vi "VD-test.vi"() -> ()   [LabVIEW 2020, in "VD-LV-LiteVNA.lvclass"]
uses:
  VD-LV-LiteVNA.lvclass
  VD-settings.ctl
  VD-data_req.ctl
  hardware-protocol/serial/HP-S-data.ctl
  VD-device_info.ctl
  VD-connection_settings.ctl
  hardware-protocol/serial/HP-S-baudrate.ctl
  VD-session_info.ctl
  VD-data_read_status.ctl
  VD-settings_status.ctl
  VD-settingsEasy.ctl
  VD-sampleSize.ctl
  VD-LV-LiteVNA.lvclass/VD-LV-LiteVNA.ctl
  hardware-protocol/serial/HP-S-Serial.lvclass
panel:
  out "current time":timestamp
  in  "Tab Control":enum32{"Main", "Bonus"}(tab)
  in  "Set Settings":bool
  in  "Settings":T1
  out "Settings status":T2
  in  "Set Settings easy":bool
  in  "settings":T3={"Start [hz]"=1000000, "Stop [hz]"=5000000, "sampleSize"=101} {"sampleSize" items=["101"=101, "201"=201, "401"=401, "601"=601, "801"=801, "1001"=1001]; "Stop [hz]" format="%.0p"; "Start [hz]" format="%.0p"}
  in  "Get Settings":bool
  in  "Get Data":bool
  in  "data req":T5
  out "read buffer":T6 format="%x"
  out "size(s)":i32
  in  "get device settings":bool
  out "device info":T7
  in  "raw request":bool
  in  "raw write buffer":T6 format="%x"
  out "read bufferraw":T6 format="%x"
  out "size(s) raw":i32
  in  "read back?":bool
  out "Get Settings status":T2
  out "data status":T8
  out "Valid Data?":bool
  out "size":i32
  out "XY Graph":cluster{u64[], dbl[]}[](graph)
  in  "get set":bool
  out "session info":T9 {"last get" format="%x"; "last set" format="%x"}
  out "Remaining Bytes":u32
  out "Emtpied size(s)":i32
  out "Emtpied buffer":T6 format="%x"
  in  "Empty Buffer":bool
  out "error IO":errorcluster
  in  "connection settings":T10={"Com"="", "baud rate (9600)"=38400} {"baud rate (9600)" items=["75"=75, "110"=110, "134"=134, "150"=150, "300"=300, "600"=600, "1200"=1200, "1800"=1800, "2400"=2400, "4800"=4800, "7200"=7200, "9600"=9600, "14400"=14400, "19200"=19200, "28800"=28800, "38400"=38400, "56000"=56000, "57600"=57600, "115200"=115200, "128000"=128000, "230400"=230400]}
  out "error out":errorcluster
  in  "Free Run":bool
  in  "Disconnect":bool
  in  "Stop":bool
  in  "Connect":bool
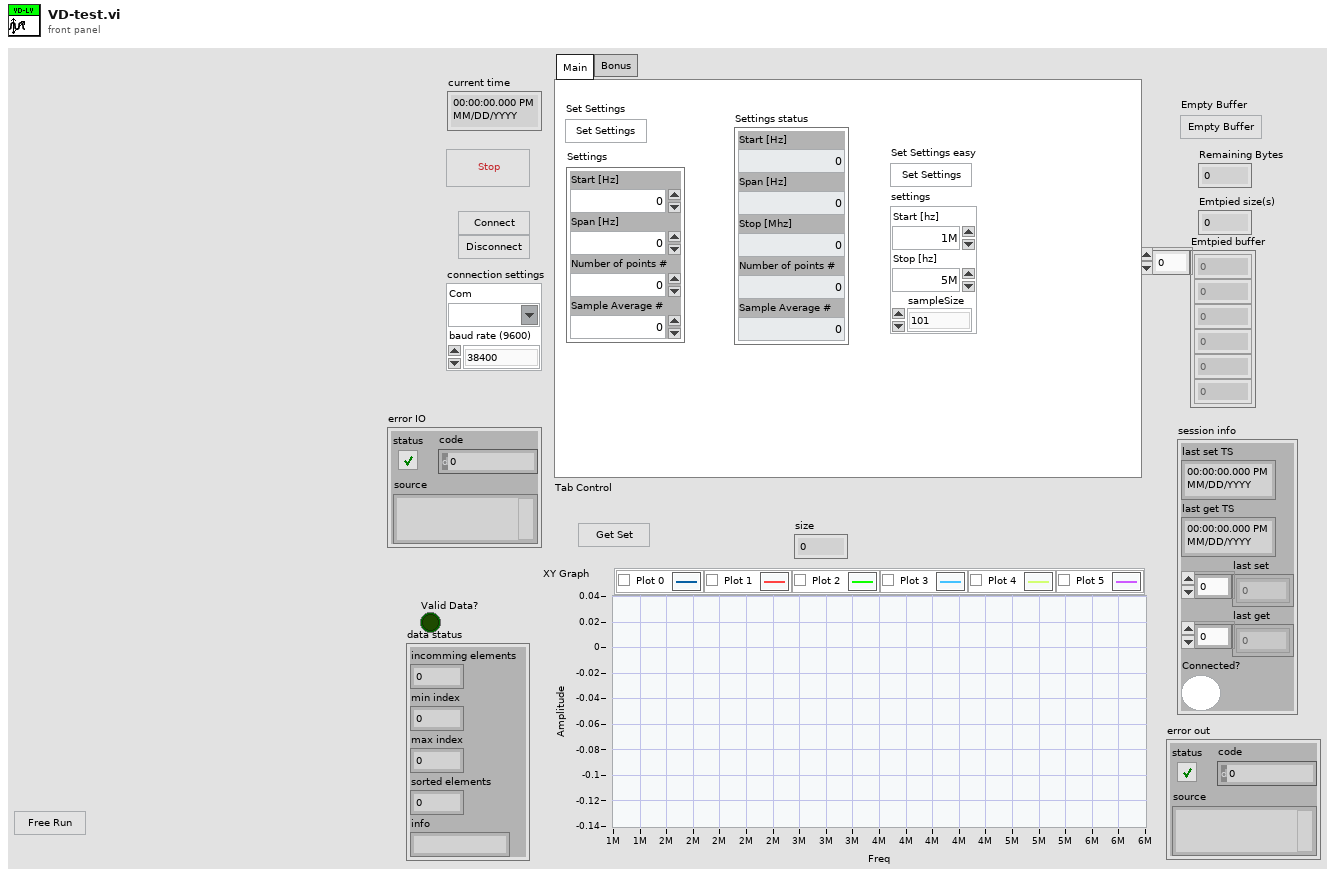
[diagram p1: front panel]
types:
  T1 = typedef "VD-LV-LiteVNA.lvclass/VD-settings.ctl" = cluster{"Start [Hz]":u64, "Span [Hz]":u64, "Number of points #":u16, "Sample Average #":u16}
  T2 = typedef "VD-LV-LiteVNA.lvclass/VD-settings_status.ctl" = cluster{"Start [Hz]":u64, "Span [Hz]":u64, "Stop [Mhz]":u64, "Number of points #":u16, "Sample Average #":u16}
  T3 = typedef "VD-LV-LiteVNA.lvclass/VD-settingsEasy.ctl" = cluster{"Start [hz]":u64, "Stop [hz]":u64, "sampleSize":T4}
  T4 = typedef "VD-LV-LiteVNA.lvclass/VD-sampleSize.ctl" = u16
  T5 = typedef "VD-LV-LiteVNA.lvclass/VD-data_req.ctl" = cluster{"datasize":u8}
  T6 = typedef "HP-S-Serial.lvclass/HP-S-data.ctl" = u8[]
  T7 = typedef "VD-LV-LiteVNA.lvclass/VD-device_info.ctl" = cluster{"ID":u8}
  T8 = typedef "VD-LV-LiteVNA.lvclass/VD-data_read_status.ctl" = cluster{"incomming elements":i32, "min index":u16, "max index":u16, "sorted elements":i32, "info":string}
  T9 = typedef "VD-LV-LiteVNA.lvclass/VD-session_info.ctl" = cluster{"last set TS":timestamp, "last get TS":timestamp, "last set":T6, "last get":T6, "Connected?":bool}
  T10 = typedef "VD-LV-LiteVNA.lvclass/VD-connection_settings.ctl" = cluster{"Com":refnum<visa-resource-name>, "baud rate (9600)":T11}
  T11 = typedef "HP-S-Serial.lvclass/HP-S-baudrate.ctl" = u32
  T12 = typedef "VD-LV-LiteVNA.lvclass/VD-VNA_data.ctl" = cluster{"S1":cdb[], "S11":cdb[], "S21":cdb[], "Frequency":u64[]}
  T13 = typedef "VD-LV-LiteVNA.lvclass/VD-graph_data.ctl" = cluster{u64[], dbl[]}[]
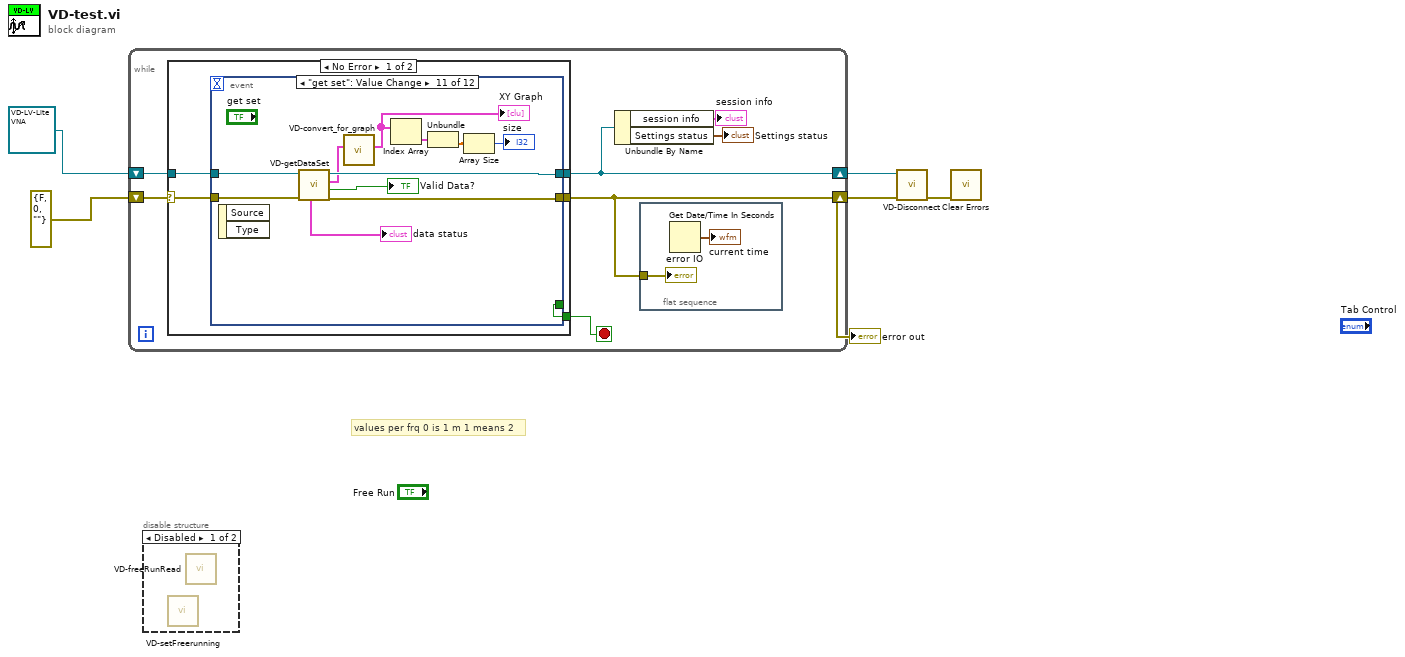
[diagram p0: block diagram]
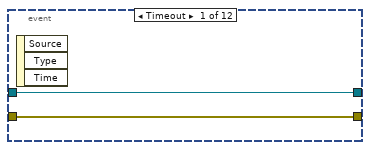
[diagram p2: hidden frame]
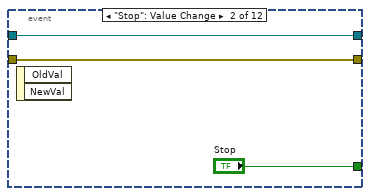
[diagram p3: hidden frame]
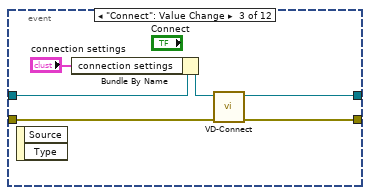
[diagram p4: hidden frame]
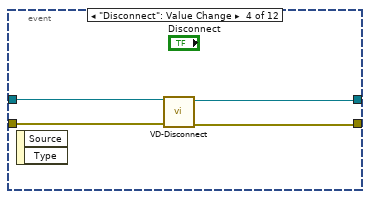
[diagram p5: hidden frame]
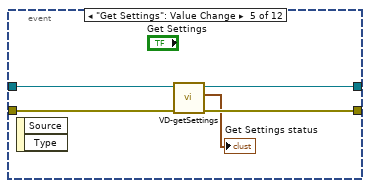
[diagram p6: hidden frame]
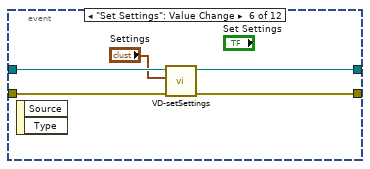
[diagram p7: hidden frame]
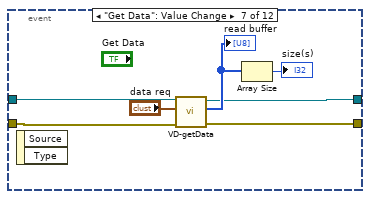
[diagram p8: hidden frame]
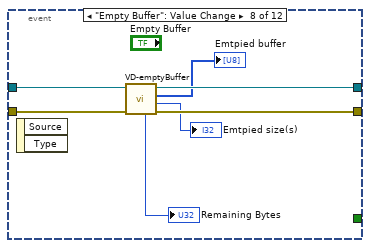
[diagram p9: hidden frame]
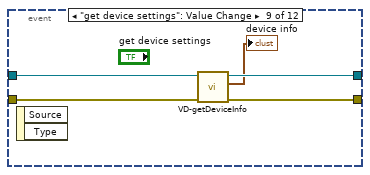
[diagram p10: hidden frame]
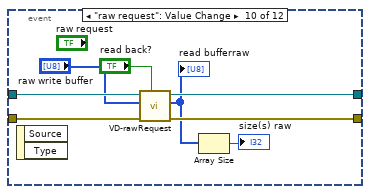
[diagram p11: hidden frame]
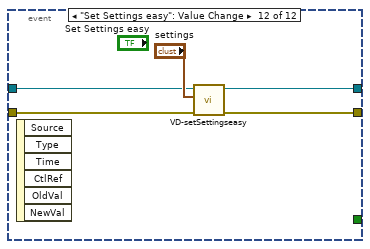
[diagram p12: hidden frame]
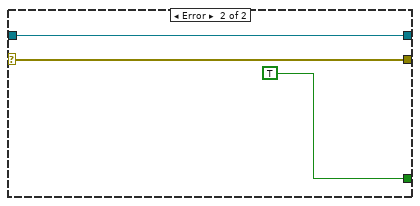
[diagram p13: hidden frame]
diagram:
  # "values per frq 0 is 1 m 1 means 2"
  n1 = while {
    shift-right: [w10] -> w3
    shift-left: errorcluster {"status"=FALSE, "code"=0, "source"=""} ("error IO") -> [w11]
    shift-right: [w8] -> w2
    shift-left: refnum<class "VD-LV-LiteVNA.lvclass"> refnum ("VD-LV-LiteVNA out") -> [w9]
    stop <- w12 stop-if-true
    n2 = case shown="No Error" w11 {
      selector: w11 -> [w19 w88]
      tunnel: [w17 TRUE] -> w12
      tunnel: [w18 w88] -> w10
      tunnel: w9 -> [w16 w89]
      tunnel: [w15 w89] -> w8
      frame No Error {
        n3 = event shown="[10] \"get set\": Value Change" {
          selector: _ -> [_ _ _ _ _ _ _ _ _ _ _ _]
          dyn-events: _ -> [_ _ _ _ _ _ _ _ _ _ _ _]
          timeout: _ -> [_ _ _ _ _ _ _ _ _ _ _ _]
          tunnel: w19 -> [w21 w23 w30 w33 w39 w43 w50 w57 w62 w70 w81 w85]
          tunnel: [w21 w23 w27 w32 w36 w41 w45 w56 w61 w67 w80 w83] -> w18
          tunnel: [_ "Stop" _ _ _ _ _ _ _ _ _ _] -> w17
          tunnel: w16 -> [w20 w22 w29 w34 w38 w44 w51 w58 w63 w71 w82 w86]
          tunnel: [w20 w22 w28 w31 w37 w42 w46 w55 w60 w68 w79 w84] -> w15
          event Timeout {
            n4 = event-data() -> ()  [unwired: 1 in, 3 out]
          }
          event "Stop": Value Change {
            n5 = event-data() -> ()  [unwired: 1 in, 2 out]
          }
          event "Connect": Value Change {
            n6 = event-data() -> ()  [unwired: 1 in, 2 out]
            n7 = Bundle By Name(cluster=w29, "connection settings"="connection settings") -> (w26:refnum<class "VD-LV-LiteVNA.lvclass">)
            n8 = call-dynamic "VD-Connect.vi"("error in (no error)"=w30, "VD-LV-LiteVNA in"=w26) -> ("error out"=w27:errorcluster, "VD-LV-LiteVNA out"=w28:refnum<class "VD-LV-LiteVNA.lvclass">)  [unwired: 8 in]
          }
          event "Disconnect": Value Change {
            n9 = event-data() -> ()  [unwired: 1 in, 2 out]
            n10 = call-dynamic "VD-Disconnect.vi"("error in (no error)"=w33, "VD-LV-LiteVNA in"=w34) -> ("error out"=w32:errorcluster, "VD-LV-LiteVNA out"=w31:refnum<class "VD-LV-LiteVNA.lvclass">)  [unwired: 8 in]
          }
          event "Get Settings": Value Change {
            n11 = event-data() -> ()  [unwired: 1 in, 2 out]
            n12 = call "VD-getSettings.vi"("error in (no error)"=w39, "VD-LV-LiteVNA in"=w38) -> ("error out"=w36:errorcluster, "Settings status"=→"Get Settings status":T2, "VD-LV-LiteVNA out"=w37:refnum<class "VD-LV-LiteVNA.lvclass">)  [unwired: 7 in]
          }
          event "Set Settings": Value Change {
            n13 = event-data() -> ()  [unwired: 1 in, 2 out]
            n14 = call "VD-setSettings.vi"("error in (no error)"=w43, "Settings"="Settings", "VD-LV-LiteVNA in"=w44) -> ("error out"=w41:errorcluster, "VD-LV-LiteVNA out"=w42:refnum<class "VD-LV-LiteVNA.lvclass">)  [unwired: 7 in]
          }
          event "Get Data": Value Change {
            n15 = event-data() -> ()  [unwired: 1 in, 2 out]
            n16 = call-dynamic "VD-getData.vi"("error in (no error)"=w50, "data req"="data req", "VD-LV-LiteVNA in"=w51) -> ("error out"=w45:errorcluster, "read buffer"=w48:T6, "VD-LV-LiteVNA out"=w46:refnum<class "VD-LV-LiteVNA.lvclass">)  [unwired: 6 in]
            "read buffer" <- w48
            n17 = Array Size(array=w48) -> (size(s)=→"size(s)":i32)
          }
          event "Empty Buffer": Value Change {
            n18 = event-data() -> ()  [unwired: 1 in, 2 out]
            n19 = call-dynamic "VD-emptyBuffer.vi"("error in (no error)"=w57, "VD-LV-LiteVNA in"=w58) -> ("error out"=w56:errorcluster, "size(s)"=→"Emtpied size(s)":i32, "read buffer"=→"Emtpied buffer":T6, "VD-LV-LiteVNA out"=w55:refnum<class "VD-LV-LiteVNA.lvclass">, "Remaining Bytes at Port"=→"Remaining Bytes":u32)  [unwired: 5 in]
          }
          event "get device settings": Value Change {
            n20 = event-data() -> ()  [unwired: 1 in, 2 out]
            n21 = call "VD-getDeviceInfo.vi"("error in (no error)"=w62, "VD-LV-LiteVNA in"=w63) -> ("error out"=w61:errorcluster, "device info"=→"device info":T7, "VD-LV-LiteVNA out"=w60:refnum<class "VD-LV-LiteVNA.lvclass">)  [unwired: 7 in]
          }
          event "raw request": Value Change {
            n22 = event-data() -> ()  [unwired: 1 in, 2 out]
            n23 = call-dynamic "VD-rawRequest.vi"("read back?"="read back?", "error in (no error)"=w70, "write buffer"="raw write buffer", "VD-LV-LiteVNA in"=w71) -> ("error out"=w67:errorcluster, "read buffer"=w66:T6, "VD-LV-LiteVNA out"=w68:refnum<class "VD-LV-LiteVNA.lvclass">)  [unwired: 5 in]
            "read bufferraw" <- w66
            n24 = Array Size(array=w66) -> (size(s)=→"size(s) raw":i32)
          }
          event "get set": Value Change {
            n25 = event-data() -> ()  [unwired: 1 in, 2 out]
            n26 = call-dynamic "VD-getDataSet.vi"("error in (no error)"=w81, "VD-LV-LiteVNA in"=w82) -> ("error out"=w80:errorcluster, "Valid Data?"=→"Valid Data?":bool, "VNA data"=w73:T12, "VD-LV-LiteVNA out"=w79:refnum<class "VD-LV-LiteVNA.lvclass">, "data status"=→"data status":T8)  [unwired: 5 in]
            n27 = call "VD-convert_for_graph.vi"("VNA data"=w73) -> ("Graph Data"=w72:T13)  [unwired: 10 in]
            "XY Graph" <- w72
            n28 = Index Array(array=w72) -> (element=w78:cluster{u64[], dbl[]})  [unwired: 1 in]
            n29 = Unbundle(w78) -> (w77:dbl[])  [unwired: 1 out]
            n30 = Array Size(array=w77) -> (size(s)=→"size":i32)
          }
          event "Set Settings easy": Value Change {
            n31 = event-data() -> ()  [unwired: 1 in, 6 out]
            n32 = call "VD-setSettingseasy.vi"("error in (no error)"=w85, "settings"="settings", "VD-LV-LiteVNA in"=w86) -> ("error out"=w83:errorcluster, "VD-LV-LiteVNA out"=w84:refnum<class "VD-LV-LiteVNA.lvclass">)  [unwired: 7 in]
          }
        }
      }
      frame Error {
      }
    }
    n33 = Unbundle By Name(w8) -> ("session info"=→"session info":T9, "Settings status"=→"Settings status":T2)
    n34 = flat-sequence {
      tunnel: w10 -> [w14]
      frame #0 {
        n35 = Get Date/Time In Seconds() -> (seconds since 1Jan1904=→"current time":timestamp)
        "error IO" <- w14
      }
    }
  }
  "error out" <- w3
  n36 = disable-structure shown="Disabled" {
    frame Disabled {
      n37 = call-dynamic "VD-setFreerunning.vi"() -> ()  [unwired: 10 in, 2 out]
      n38 = call-dynamic "VD-freeRunRead.vi"() -> ()  [unwired: 10 in, 2 out]
    }
    frame Enabled {
    }
  }
  n39 = call-dynamic "VD-Disconnect.vi"("error in (no error)"=w3, "VD-LV-LiteVNA in"=w2) -> ("error out"=w1:errorcluster)  [unwired: 8 in, 1 out]
  n40 = call <vilib>:"Clear Errors.vi"("error in (no error)"=w1) -> ()  [unwired: 5 in, 2 out]
